vi "Channels.vi"() -> ()   [LabVIEW 2012]
panel:
  in  "Z Channel":tag="Dev1/ao3"
  in  "Laser voltage":tag="Dev1/ao2"
  in  "HoldChannel.exe":path=path "C:/Users/Loncar/Desktop/ESR VIs - Srujan/Sam Kim/PB/HoldChannel.exe"
  in  "spinapi.dll":path=path "C:/SpinCore/SpinAPI/dll/spinapi64.dll"
  in  "Sample clock line":tag="/Dev1/PFI9" caption="Sample clock"
  in  "Y Channel":tag="Dev1/ao1"
  in  "X Channel":tag="Dev1/ao0"
  in  "Counter(s)":tag="Dev1/ctr0" caption="Counter"
  # "(X)"
  # "(Z)"
  # "(Y)"
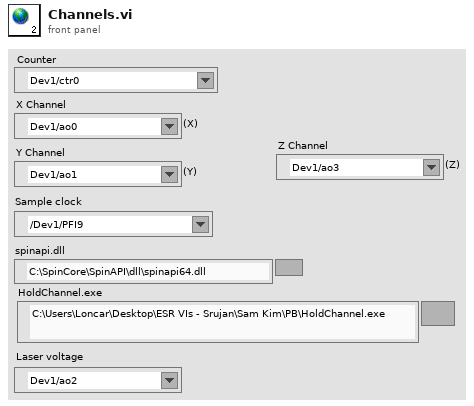
[diagram p1: front panel]
diagram:
